vi "Vector2DRotate.vi"(0 "Vector":T1, 3 "Theta":dbl) -> (7 "Rotated Vector":T1)   [LabVIEW 2018]
uses:
  Vector2D.ctl
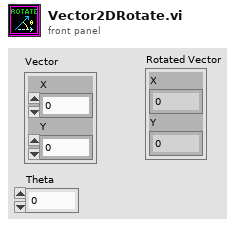
[diagram p1: front panel]
types:
  T1 = typedef "Vector2D.ctl" = cluster{"X":dbl, "Y":dbl}
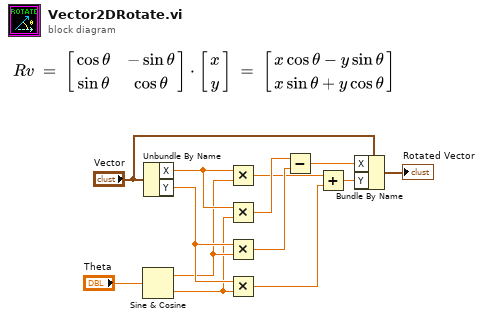
[diagram p0: block diagram]
diagram:
  n1 = Sine & Cosine(0:"Theta") -> (1:w8:dbl, 2:w7:dbl)
  n2 = Unbundle By Name("Vector") -> ("X"=w10:dbl, "Y"=w9:dbl)
  n3 = Multiply(x=w10, y=w8) -> (x*y=w2:dbl)
  n4 = Multiply(x=w10, y=w7) -> (x*y=w5:dbl)
  n5 = Multiply(x=w9, y=w8) -> (x*y=w4:dbl)
  n6 = Multiply(x=w9, y=w7) -> (x*y=w1:dbl)
  n7 = Subtract(x=w5, y=w4) -> (x-y=w6:dbl)
  n8 = Add(x=w2, y=w1) -> (x+y=w3:dbl)
  n9 = Bundle By Name(cluster="Vector", "X"=w6, "Y"=w3) -> (→"Rotated Vector":T1)
